vi "Obtain Module and Vi Name From User Event Name.vi"(7 "Mode":T1=enum."Request", 11 "User Event Name":string) -> (2 "Vi":string, 3 "Module":string)   [LabVIEW 2021, in "TAF Proj Document Type.lvlib" / "Project Parser.lvlib"]
uses:
  <vilib>/Wovalab/AntiDoc/Document Type/Add-ons/LabVIEW TAF Project/Project Parser/Project Parser.lvlib
  <vilib>/Wovalab/AntiDoc/Document Type/Add-ons/LabVIEW TAF Project/Project Parser/Module Fonctions--enum.ctl
  <vilib>/Wovalab/AntiDoc/Document Type/Add-ons/LabVIEW TAF Project/TAF Proj Document Type.lvlib
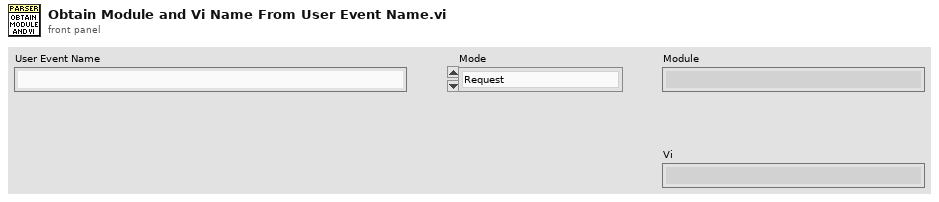
[diagram p1: front panel]
types:
  T1 = typedef "TAF Proj Document Type.lvlib/Project Parser.lvlib/Module Fonctions--enum.ctl" = enum16{"Event Registration", "Request"}
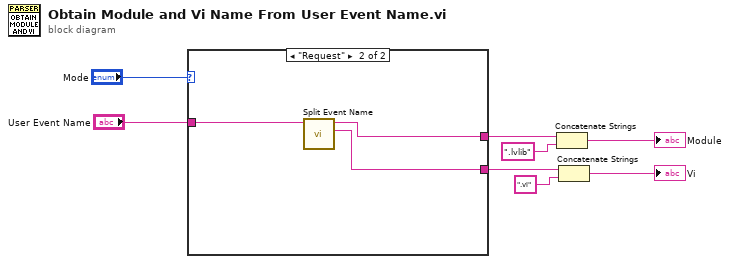
[diagram p0: block diagram]
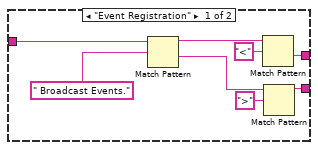
[diagram p2: hidden frame]
diagram:
  n1 = case shown="\"Request\"" "Mode" {
    tunnel: "User Event Name" -> [w16 w19]
    tunnel: [w15 w17] -> w5
    tunnel: [w14 w18] -> w3
    frame "Event Registration" {
      n2 = Match Pattern(string=w16, regular expression=" Broadcast Events.") -> (before substring=w10:string, after substring=w13:string)  [unwired: 1 in, 2 out]
      n3 = Match Pattern(string=w10, regular expression="<") -> (after substring=w14:string)  [unwired: 1 in, 3 out]
      n4 = Match Pattern(string=w13, regular expression=">") -> (before substring=w15:string)  [unwired: 1 in, 3 out]
    }
    frame "Request" {
      n5 = call <vilib>:"Split Event Name.vi"("Event Name"=w19) -> ("Vi Name"=w17:string, "Library Name"=w18:string)  [unwired: 8 in, 1 out]
    }
  }
  n6 = Concatenate Strings(w3, ".lvlib" ("string")) -> (→"Module":string)
  n7 = Concatenate Strings(w5, ".vi" ("string")) -> (→"Vi":string)
